vi "ExSubFullYBin.vi"(2 "error in (no error)":errorcluster, 3 "Camera Handle":u32) -> (0 "error out":errorcluster, 1 "Camera Handle":u32)   [LabVIEW 2010]
panel:
  # "ExSubFullYBin:\nThis sub-vi gets the camera dimensions\nand picks/programs the center strip/row \nas an ROI."
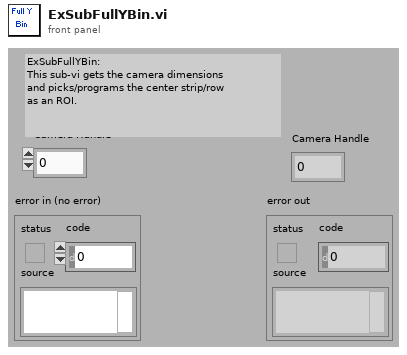
[diagram p1: front panel]
types:
  T1 = cluster{"X start":u32, "X end":u32, "X Binning/Grouping":u32, "Y start":u32, "Y end":u32, "Y Binning/Grouping":u32}
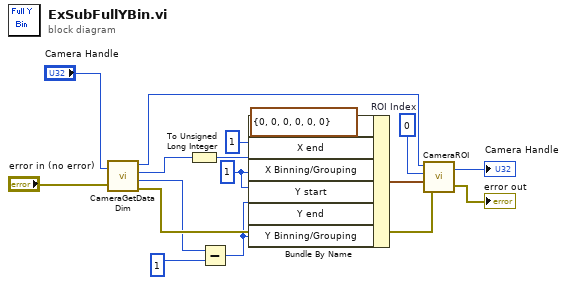
[diagram p0: block diagram]
diagram:
  w5 = u32 0  # ROI Index
  w4 = u32 1
  n1 = call <userlib>:"CameraGetDataDim.vi"("Camera Handle"="Camera Handle", "error in"="error in (no error)") -> ("Camera Handle"=w15:u32, "Xdim"=w12:u32, "Ydim"=w2:u32, "error out"=w13:errorcluster)
  n2 = To Unsigned Long Integer(number=w12) -> (unsigned 32bit integer=w8:u32)
  n3 = Subtract(x=w2, y=1) -> (x-y=w1:u32)
  n4 = Bundle By Name(cluster=T1 {"X start"=0, "X end"=0, "X Binning/Grouping"=0, "Y start"=0, "Y end"=0, "Y Binning/Grouping"=0} ("ROI Params"), "X start"=u32 1, "X end"=w8, "X Binning/Grouping"=w4, "Y start"=w4, "Y end"=w1, "Y Binning/Grouping"=w1) -> (w7:T1)
  n5 = call <userlib>:"CameraROI.vi"("error in"=w13, "ROI Params"=w7, "ROI Index"=w5, "Camera Handle"=w15) -> ("error out"=→"error out":errorcluster, "Camera Handle"=→"Camera Handle":u32)
